vi "GraphPanelResize.vi"(8 "error in (no error)":errorcluster caption="entrée d'erreur (pas d'erreur)", 11 "Interface en entrée":refnum<class "Interface.lvclass"> caption="DNL_LabVIEW Object in") -> (0 "error out":errorcluster caption="sortie d'erreur", 3 "Interface en sortie":refnum<class "Interface.lvclass"> caption="DNL_LabVIEW Object out")   [LabVIEW 2010, in "Interface.lvclass"]
uses:
  Interface.lvclass
  Interface.lvclass/Interface.ctl
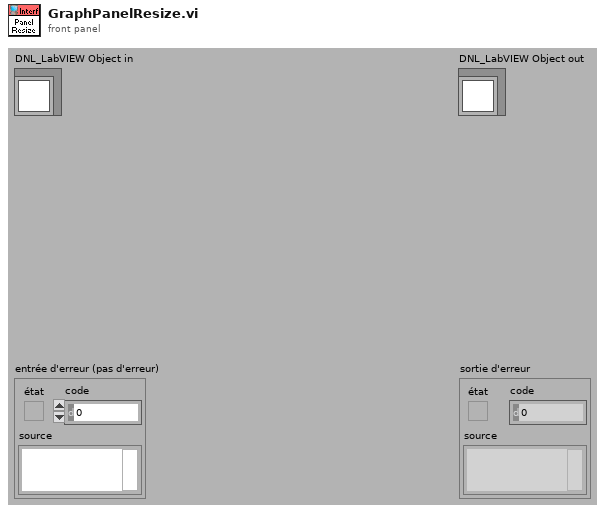
[diagram p1: front panel]
types:
  T1 = typedef "LVRectTypeDef.ctl" = cluster{"left":i16, "top":i16, "right":i16, "bottom":i16}
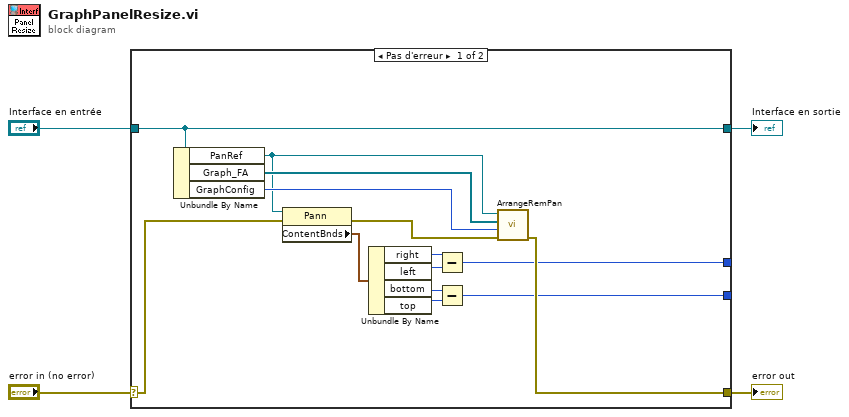
[diagram p0: block diagram]
diagram:
  n1 = case shown="Pas d'erreur" "error in (no error)" {
    selector: "error in (no error)" -> [w13 w20]
    tunnel: [w15 w20] -> w3
    tunnel: [w18 w19] -> w1
    tunnel: "Interface en entrée" -> [w18 w19]
    tunnel: [w6 _] -> _
    tunnel: [w5 _] -> _
    frame No Error {
      n2 = Unbundle By Name(w18) -> ("PanRef"=w14:refnum<vi>, "Graph_FA"=w17:refnum<vi>[], "GraphConfig"=w16:u32)
      n3 = property class="Pann"(reference=w14, error in=w13) -> (error out=w7:errorcluster, "ContentBnds"=w8:T1)  [unwired: 1 out]
      n4 = Unbundle By Name(w8) -> ("right"=w9:i16, "left"=w10:i16, "bottom"=w12:i16, "top"=w11:i16)
      n5 = Subtract(x=w9, y=w10) -> (x-y=w6:i16)
      n6 = Subtract(x=w12, y=w11) -> (x-y=w5:i16)
      n7 = call "ArrangeRemPan.vi"("error in (no error)"=w7, "Configuration"=w16, "FARefArr"=w17, "PanRef"=w14) -> ("error out"=w15:errorcluster)  [unwired: 5 in, 2 out]
    }
    frame Error {
    }
  }
  "error out" <- w3
  "Interface en sortie" <- w1
